vi "梦幻城堡C6~20通信.vi"() -> ()   [LabVIEW 2016, in "环境动力监测库.lvlib" / "UPS库.lvlib"]
uses:
  <vilib>/Instr/_visa.llb/VISA Configure Serial Port (Instr).vi
  <vilib>/Utility/config.llb/NI_LVConfig.lvlib
  <vilib>/ptbypt/NI_PtbyPt.lvlib
panel:
  out "Status-WA":T1
  out "Status-Q6":T2
  in  "open":bool
  in  "close":bool
  out "通信指示":bool
  in  "关机":bool
  in  "功率查询":bool
  in  "状态查询":bool
  out "读取缓冲区":string
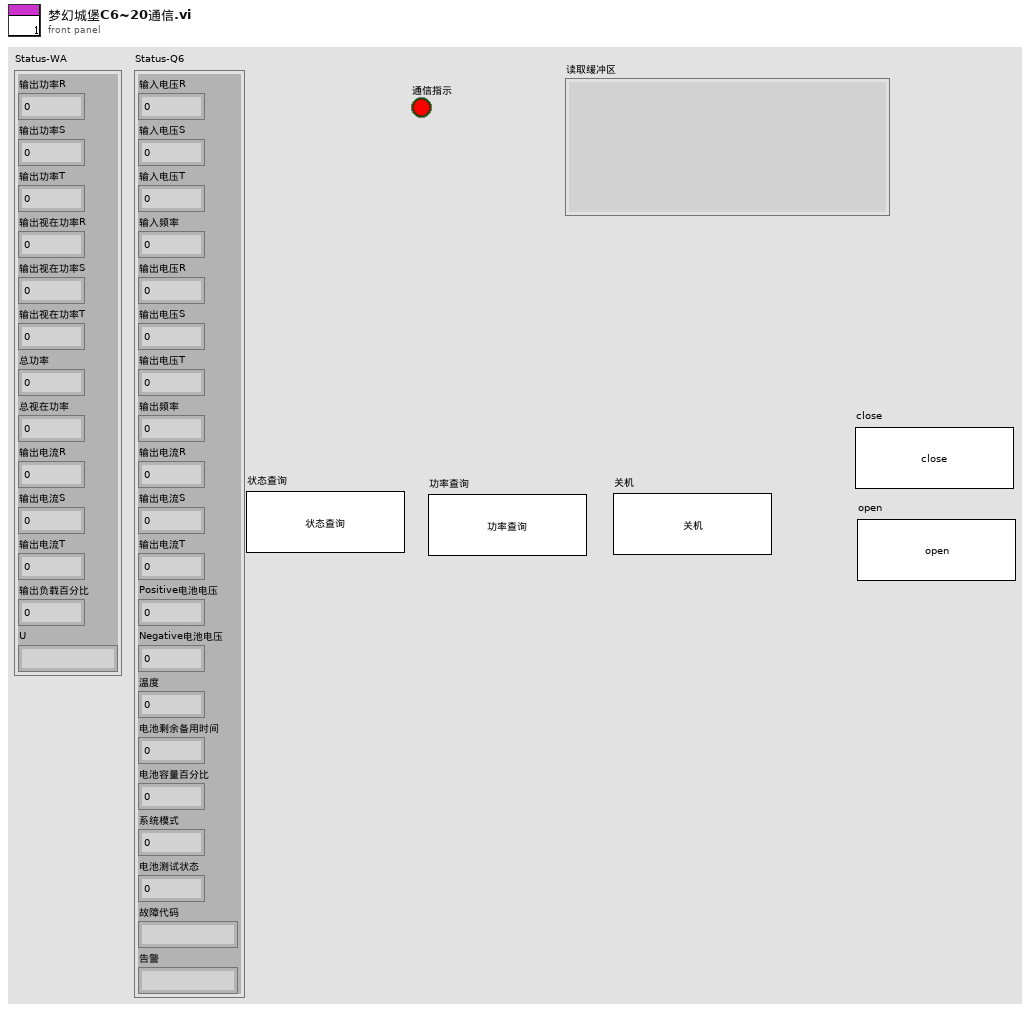
[diagram p1: front panel]
types:
  T1 = cluster{"输出功率R":dbl, "输出功率S":dbl, "输出功率T":dbl, "输出视在功率R":dbl, "输出视在功率S":dbl, "输出视在功率T":dbl, "总功率":dbl, "总视在功率":dbl, "输出电流R":dbl, "输出电流S":dbl, "输出电流T":dbl, "输出负载百分比":dbl, "U":string}
  T2 = cluster{"输入电压R":dbl, "输入电压S":dbl, "输入电压T":dbl, "输入频率":dbl, "输出电压R":dbl, "输出电压S":dbl, "输出电压T":dbl, "输出频率":dbl, "输出电流R":dbl, "输出电流S":dbl, "输出电流T":dbl, "Positive电池电压":dbl, "Negative电池电压":dbl, "温度":dbl, "电池剩余备用时间":dbl, "电池容量百分比":dbl, "系统模式":dbl, "电池测试状态":dbl, "故障代码":string, "告警":string}
  T3 = cluster{"枚举":enum16{"open", "read", "write", "close"}, "写入缓冲区":string}
  T4 = typedef "NI_LVConfig.lvlib/Config Data RefNum.ctl" = refnum<k1>
  T5 = cluster{"baud rate (9600)":u32, "stop bits (10: 1 bit)":u16, "parity (0:none)":enum16{"None", "Odd", "Even", "Mark", "Space"}, "data bits (8)":u16, "timeout (10sec)":u32}
  T6 = cluster{"漏水监测输出":bool, "门禁监测输出":bool, "温湿度监测输出":bool, "烟雾监测输出":bool, "空调监测输出":bool, "自动重合闸输出":bool, "红外入侵输出":bool, "振动输出":bool, "UPS输出":bool, "蓄电池输出":bool}
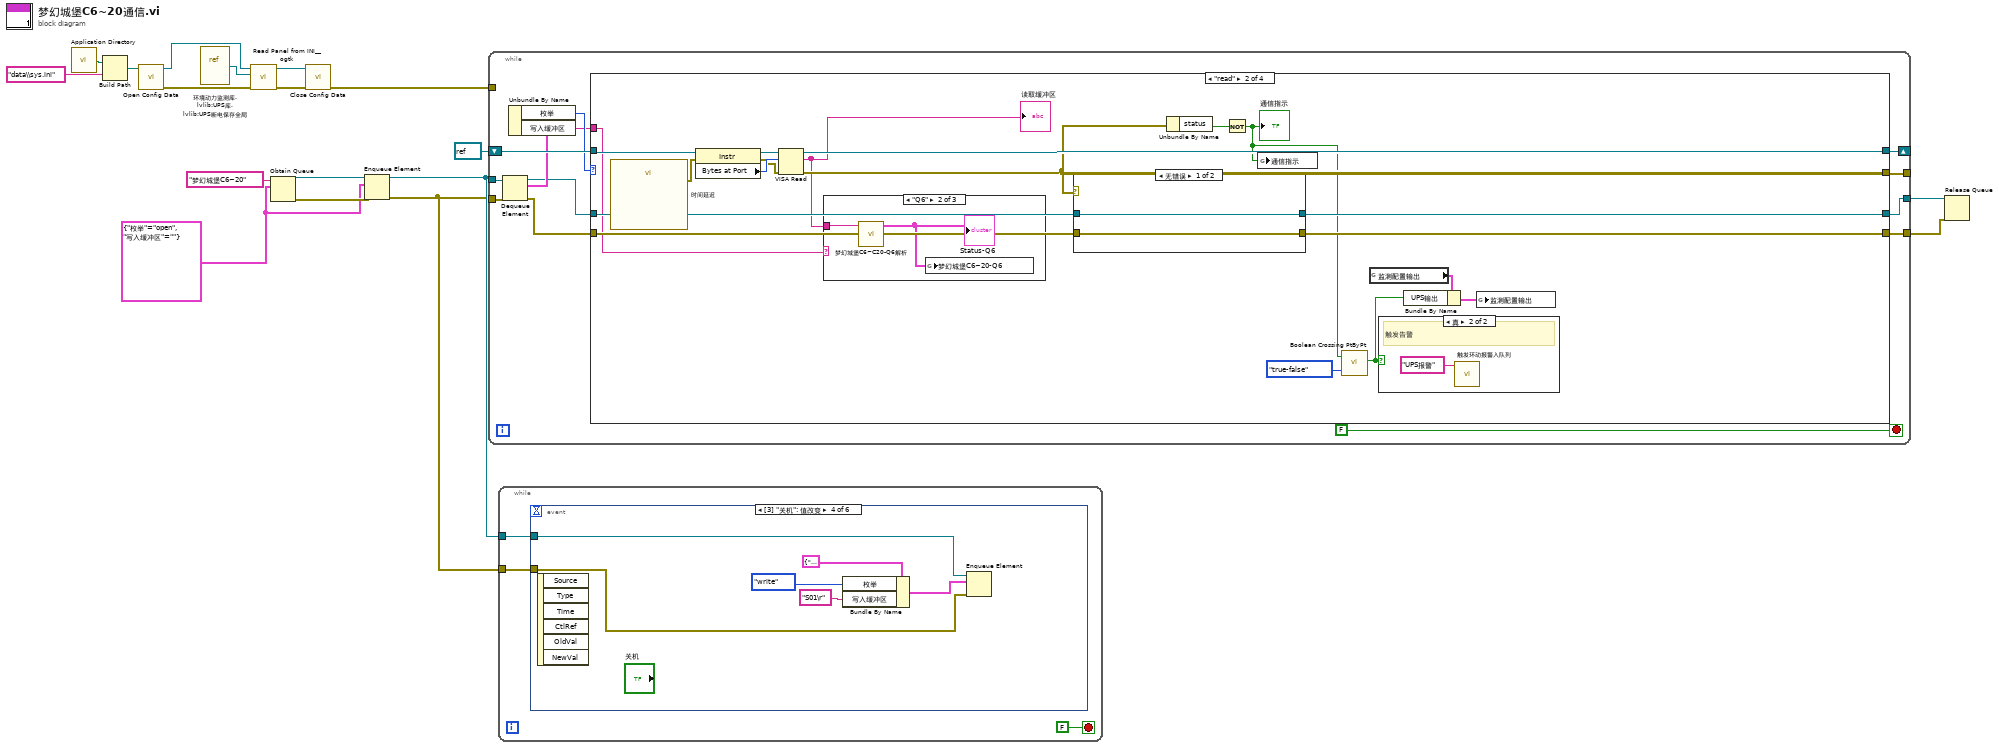
[diagram p0: block diagram]
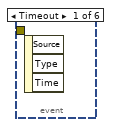
[diagram p2: hidden frame]
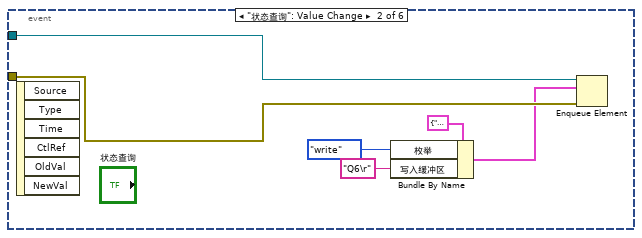
[diagram p3: hidden frame]
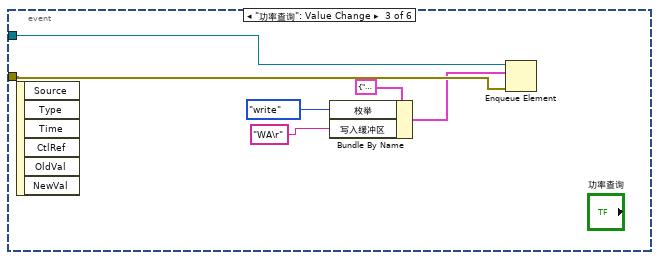
[diagram p4: hidden frame]
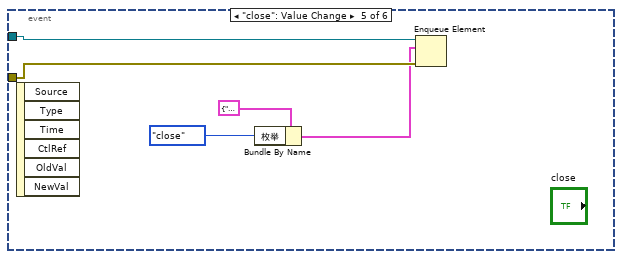
[diagram p5: hidden frame]
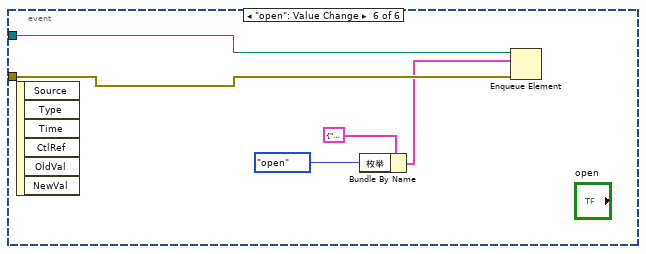
[diagram p6: hidden frame]
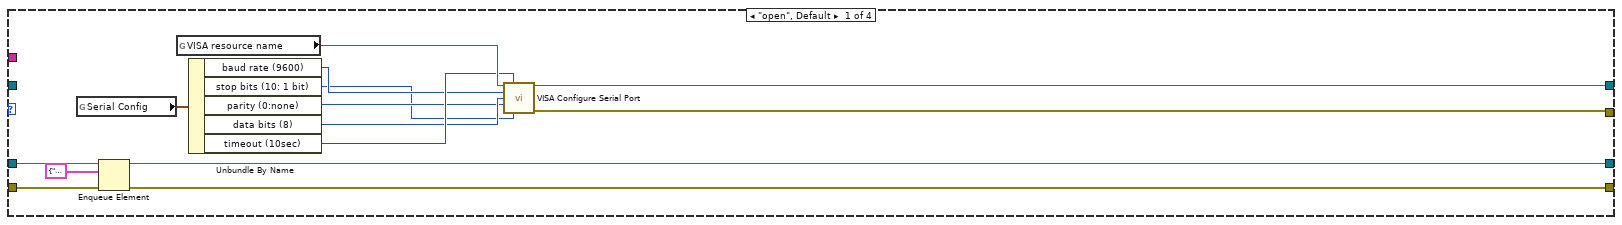
[diagram p7: hidden frame]
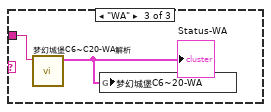
[diagram p10: hidden frame]
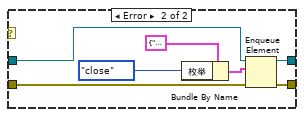
[diagram p11: hidden frame]
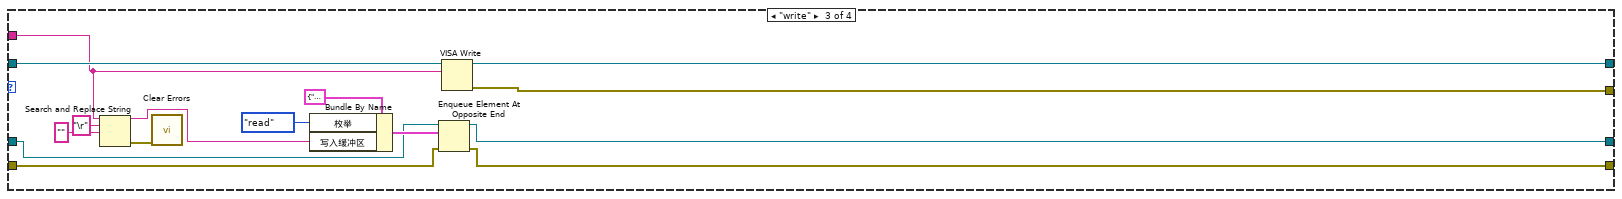
[diagram p12: hidden frame]
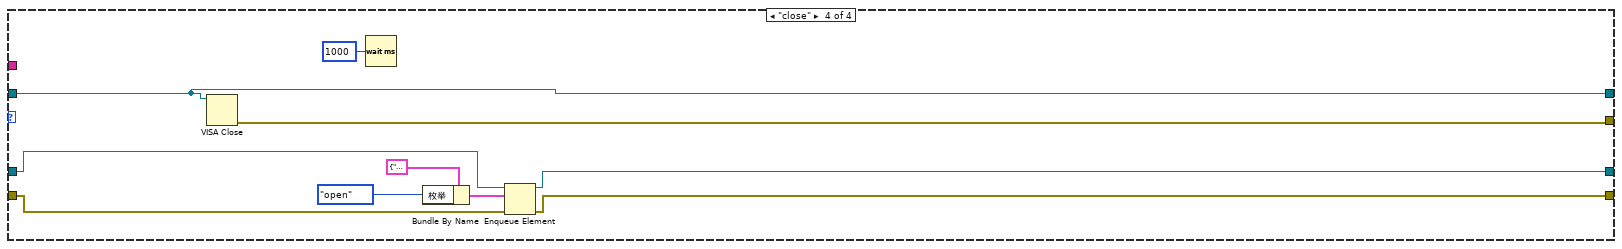
[diagram p13: hidden frame]
diagram:
  w13 = T3 {"枚举"=enum."open", "写入缓冲区"=""}
  n1 = call <vilib>:"Application Directory.vi"() -> ("Application Directory"=w9:path)
  n2 = Build Path(base path=w9, name or relative path="data\\sys.ini" ("名称或相对路径")) -> (appended path=w7:path)
  n3 = call <vilib>:"Open Config Data.vi"("configuration file path"=w7) -> ("error out"=w3:errorcluster, "refnum"=w6:T4)  [unwired: 8 in, 1 out]
  n4 = vi-ref "环境动力监测库.lvlib:UPS库.lvlib:UPS断电保存全局.vi"() -> (w5:refnum<vi>)
  n5 = call <userlib>:"Read Panel from INI__ogtk.vi"("error in (no error)"=w3, "VI ref"=w5, "refnum"=w6) -> ("error out"=w2:errorcluster, "refnum out"=w4:T4)  [unwired: 7 in]
  n6 = Obtain Queue(name (unnamed)="梦幻城堡C6~20" ("名称（未命名）"), element data type=w13) -> (queue out=w17:refnum<queue>, error out=w16:errorcluster)  [unwired: 3 in, 1 out]
  n7 = call <vilib>:"Close Config Data.vi"("error in (no error)"=w2, "refnum"=w4) -> ("error out"=w1:errorcluster)  [unwired: 8 in, 1 out]
  n8 = Enqueue Element(queue=w17, element=w13, error in (no error)=w16) -> (queue out=w15:refnum<queue>, error out=w14:errorcluster)  [unwired: 1 in, 1 out]
  n9 = while {
    shift-right: [w31] -> _
    shift-left: refnum<visa-resource-name> refnum ("VISA resource name out") -> [w30]
    tunnel: [w29] -> _
    tunnel: w15 -> [w27]
    tunnel: w14 -> [w26]
    tunnel: [w21] -> w11
    tunnel: [w20] -> w10
    tunnel: w1 -> [_]
    stop <- FALSE stop-if-true
    n10 = Dequeue Element(queue=w27, error in (no error)=w26) -> (queue out=w23:refnum<queue>, element=w25:T3, error out=w22:errorcluster)  [unwired: 1 in, 1 out]
    n11 = Unbundle By Name(w25) -> ("枚举"=w24:enum16{"open", "read", "write", "close"}, "写入缓冲区"=w19:string)
    n12 = case shown="\"read\"" w24 {
      tunnel: [w45 w61 w92 w102] -> w31
      tunnel: w30 -> [_ w64 w93 w102]
      tunnel: [w44 w58 w91 w103] -> w29
      tunnel: w23 -> [w35 w57 w84 w98]
      tunnel: w22 -> [w34 w56 w83 w97]
      tunnel: [w33 w55 w82 w96] -> w21
      tunnel: [w32 w54 w81 w95] -> w20
      tunnel: w19 -> [_ w53 w79 _]
      frame "open", Default {
        n13 = global read "UPS断电保存全局.vi" "Serial Config"() -> (w43:T5)
        n14 = Enqueue Element(queue=w35, element=T3 {"枚举"=enum."read", "写入缓冲区"=""}, error in (no error)=w34) -> (queue out=w33:refnum<queue>, error out=w32:errorcluster)  [unwired: 1 in, 1 out]
        n15 = global read "UPS断电保存全局.vi" "VISA resource name"() -> (w42:refnum<visa-resource-name>)
        n16 = Unbundle By Name(w43) -> ("baud rate (9600)"=w40:u32, "stop bits (10: 1 bit)"=w37:u16, "parity (0:none)"=w38:enum16{"None", "Odd", "Even", "Mark", "Space"}, "data bits (8)"=w39:u16, "timeout (10sec)"=w41:u32)
        n17 = call-poly "VISA Configure Serial Port"("VISA resource name"=w42, "timeout (10sec)"=w41, "baud rate (9600)"=w40, "data bits (8)"=w39, "parity (0:none)"=w38, "stop bits (10: 1 bit)"=w37) -> ("VISA resource name out"=w45:refnum<visa-resource-name>, "error out"=w44:errorcluster)  [unwired: 8 in]
      }
      frame "read" {
        n18 = call "时间延迟"() -> ("error out"=w59:errorcluster)  [unwired: 11 in]
        n19 = property class="Instr"(reference=w64, error in=w59) -> (reference out=w62:refnum<visa-resource-name>, error out=w51:errorcluster, "Bytes at Port"=w63:u32)
        n20 = VISA Read(VISA resource name=w62, byte count=w63, error in (no error)=w51) -> (VISA resource name out=w61:refnum<visa-resource-name>, read buffer=w52:string, error out=w58:errorcluster)  [unwired: 1 out]
        "读取缓冲区" <- w52
        n21 = case shown="\"Q6\"" w53 {
          tunnel: w52 -> [_ w67 w69]
          frame "假", Default {
          }
          frame "Q6" {
            n22 = call "梦幻城堡C6~C20-Q6解析.vi"("读取缓冲区"=w67) -> ("Status"=w66:T2)  [unwired: 10 in]
            "Status-Q6" <- w66
            n23 = global write "UPS内部交互全局.vi" "梦幻城堡C6~20-Q6"(w66) -> ()
          }
          frame "WA" {
            n24 = call "梦幻城堡C6~C20-WA解析.vi"("读取缓冲区"=w69) -> ("Status"=w68:T1)  [unwired: 10 in]
            "Status-WA" <- w68
            n25 = global write "UPS内部交互全局.vi" "梦幻城堡C6~20-WA"(w68) -> ()
          }
        }
        n26 = case shown="无错误" w58 {
          tunnel: w57 -> [w71 w72]
          tunnel: w56 -> [w70 w75]
          tunnel: [w71 w74] -> w55
          tunnel: [w70 w73] -> w54
          frame No Error {
          }
          frame Error {
            n27 = Bundle By Name(cluster=T3 {"枚举"=enum."open", "写入缓冲区"=""}, "枚举"=enum16{"open", "read", "write", "close"}."close") -> (w77:T3)
            n28 = Enqueue Element(queue=w72, element=w77, error in (no error)=w75) -> (queue out=w74:refnum<queue>, error out=w73:errorcluster)  [unwired: 1 in, 1 out]
          }
        }
        n29 = Unbundle By Name(w58) -> ("status"=w60:bool)
        n30 = Not(x=w60) -> (.not. x?=w46:bool)
        "通信指示" <- w46
        n31 = global write "UPS内部交互全局.vi" "通信指示"(w46) -> ()
        n32 = call <vilib>:"Boolean Crossing PtByPt.vi"("direction"=enum16{"either", "false-true", "true-false"}."true-false", "input"=w46) -> ("crossing"=w47:bool)  [unwired: 1 in]
        n33 = global read "断电保存全局变量.vi" "监测配置输出"() -> (w48:T6)
        n34 = case shown="真" w47 {
          frame False {
          }
          frame True {
            # "触发告警"
            n35 = call "触发环动报警入队列.vi"("报警内容"="UPS报警") -> ()  [unwired: 11 in]
          }
        }
        n36 = Bundle By Name(cluster=w48, "UPS输出"=w47) -> (w49:T6)
        n37 = global write "断电保存全局变量.vi" "监测配置输出"(w49) -> ()
      }
      frame "write" {
        n38 = Search and Replace String(input string=w79, search string="\r" ("搜索字符串"), replace string="" ("替换字符串(\"\")")) -> (result string=w80:string, error out=w88:errorcluster)  [unwired: 5 in, 2 out]
        n39 = call <vilib>:"Clear Errors.vi"("error in (no error)"=w88) -> ()  [unwired: 5 in, 2 out]
        n40 = Bundle By Name(cluster=T3 {"枚举"=enum."open", "写入缓冲区"=""}, "枚举"=enum16{"open", "read", "write", "close"}."read", "写入缓冲区"=w80) -> (w85:T3)
        n41 = Enqueue Element At Opposite End(queue=w84, element=w85, error in (no error)=w83) -> (queue out=w82:refnum<queue>, error out=w81:errorcluster)  [unwired: 1 in, 1 out]
        n42 = VISA Write(VISA resource name=w93, write buffer=w79) -> (VISA resource name out=w92:refnum<visa-resource-name>, error out=w91:errorcluster)  [unwired: 1 in, 1 out]
      }
      frame "close" {
        n43 = VISA Close(VISA resource name=w102) -> (error out=w103:errorcluster)  [unwired: 1 in]
        n44 = Wait (ms)(milliseconds to wait=u32 1000 ("等待时间（毫秒）")) -> ()  [unwired: 1 out]
        n45 = Bundle By Name(cluster=T3 {"枚举"=enum."open", "写入缓冲区"=""}, "枚举"=enum16{"open", "read", "write", "close"}."open") -> (w99:T3)
        n46 = Enqueue Element(queue=w98, element=w99, error in (no error)=w97) -> (queue out=w96:refnum<queue>, error out=w95:errorcluster)  [unwired: 1 in, 1 out]
      }
    }
  }
  n47 = while {
    tunnel: w15 -> [w105]
    tunnel: w14 -> [w104]
    stop <- FALSE stop-if-true
    n48 = event shown="[3] \"关机\": 值改变" {
      selector: _ -> [_ _ _ _ _ _]
      dyn-events: _ -> [_ _ _ _ _ _]
      timeout: _ -> [_ _ _ _ _ _]
      tunnel: w105 -> [_ w112 w118 w124 w129 w134]
      tunnel: w104 -> [_ w111 w117 w123 w128 w133]
      event Timeout {
        n49 = event-data() -> ()  [unwired: 1 in, 3 out]
      }
      event "状态查询": Value Change {
        n50 = event-data() -> ()  [unwired: 1 in, 6 out]
        n51 = Bundle By Name(cluster=T3 {"枚举"=enum."open", "写入缓冲区"=""}, "枚举"=enum16{"open", "read", "write", "close"}."write" ("元素"), "写入缓冲区"="Q6\r") -> (w107:T3)
        n52 = Enqueue Element(queue=w112, element=w107, error in (no error)=w111) -> ()  [unwired: 1 in, 3 out]
      }
      event "功率查询": Value Change {
        n53 = event-data() -> ()  [unwired: 1 in, 6 out]
        n54 = Bundle By Name(cluster=T3 {"枚举"=enum."open", "写入缓冲区"=""}, "枚举"=enum16{"open", "read", "write", "close"}."write" ("元素"), "写入缓冲区"="WA\r") -> (w113:T3)
        n55 = Enqueue Element(queue=w118, element=w113, error in (no error)=w117) -> ()  [unwired: 1 in, 3 out]
      }
      event "关机": Value Change {
        n56 = event-data() -> ()  [unwired: 1 in, 6 out]
        n57 = Bundle By Name(cluster=T3 {"枚举"=enum."open", "写入缓冲区"=""}, "枚举"=enum16{"open", "read", "write", "close"}."write" ("元素"), "写入缓冲区"="S01\r") -> (w119:T3)
        n58 = Enqueue Element(queue=w124, element=w119, error in (no error)=w123) -> ()  [unwired: 1 in, 3 out]
      }
      event "close": Value Change {
        n59 = event-data() -> ()  [unwired: 1 in, 6 out]
        n60 = Bundle By Name(cluster=T3 {"枚举"=enum."open", "写入缓冲区"=""}, "枚举"=enum16{"open", "read", "write", "close"}."close") -> (w125:T3)
        n61 = Enqueue Element(queue=w129, element=w125, error in (no error)=w128) -> ()  [unwired: 1 in, 3 out]
      }
      event "open": Value Change {
        n62 = event-data() -> ()  [unwired: 1 in, 6 out]
        n63 = Bundle By Name(cluster=T3 {"枚举"=enum."open", "写入缓冲区"=""}, "枚举"=enum16{"open", "read", "write", "close"}."open") -> (w130:T3)
        n64 = Enqueue Element(queue=w134, element=w130, error in (no error)=w133) -> ()  [unwired: 1 in, 3 out]
      }
    }
  }
  n65 = Release Queue(queue=w11, error in (no error)=w10) -> ()  [unwired: 1 in, 3 out]
